vi "libs_loader.vi"() -> ()   [LabVIEW 2010]
uses:
  Loader.dll
panel:
  out "return type":i32
  in  "arg1":i32
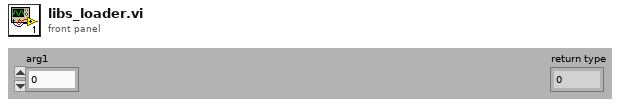
[diagram p1: front panel]
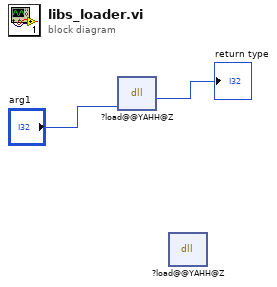
[diagram p0: block diagram]
diagram:
  n1 = dll-call lib="D:/Liakh Tanya/Dissertation/Complex/src/Loader.dll" fn="?load@@YAHH@Z"("arg1"="arg1") -> ("return type"=→"return type":i32)  [unwired: 4 in, 2 out]
  n2 = dll-call lib="D:/Liakh Tanya/Dissertation/Complex/src/Loader.dll" fn="?load@@YAHH@Z"() -> ()  [unwired: 6 in, 2 out]
